vi "Respond.vi"(7 "Sender is Waiting?(F)":bool, 8 "error in (no error)":errorcluster, 9 "Data":refnum<class "Data.lvclass">, 10 "Actor in":refnum<class "Actor.lvclass">, 11 "Request Reply Core in":refnum<class "Request Reply Core.lvclass">) -> (0 "error out":errorcluster, 2 "Actor out":refnum<class "Actor.lvclass">)   [LabVIEW 2020, in "Publisher.lvlib" / "Request Reply Core.lvclass"]
doc: "Handle the Data Action response.\n\nThe default drops the response core and does nothing else."
uses:
  Request Reply Core.lvclass
  PPL/HDH.Data.Generic.lvlibp/Data.lvclass
  PPL/HDH.Actor Framework.Core.Actor.lvlibp/1abvi3w/vi.lib/ActorFramework/Actor/Actor.lvclass
  Request Reply Core.lvclass/Request Reply Core.ctl
  Data/Request Data/Request Data.lvclass/Request Data.ctl
  Data Msg/Data Msg.lvclass/Data Msg.ctl
  Publisher Messages/Addressed Msg/Addressed Msg.lvclass/Addressed Msg.ctl
  Data/Request Data/Request Data.lvclass
  C:/Current projects/WS/PPL/HDH.Data.Generic.lvlibp/Data.lvclass
  Data Msg/Data Msg.lvclass
  C:/Current projects/WS/PPL/HDH.Actor Framework.Core.Actor.lvlibp/1abvi3w/vi.lib/ActorFramework/Message/Message.lvclass
  Publisher Messages/Addressed Msg/Addressed Msg.lvclass
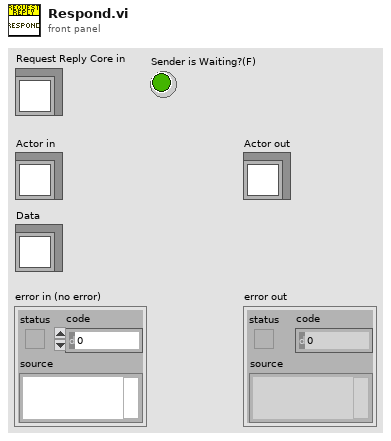
[diagram p1: front panel]
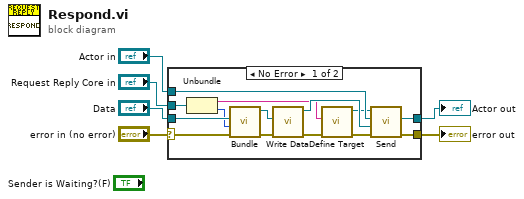
[diagram p0: block diagram]
diagram:
  n1 = case shown="No Error" "error in (no error)" {
    selector: "error in (no error)" -> [w17 w22]
    tunnel: "Request Reply Core in" -> [w20 _]
    tunnel: [w7 w22] -> w4
    tunnel: [w15 w21] -> w3
    tunnel: "Actor in" -> [w16 w21]
    tunnel: "Data" -> [w19 _]
    frame No Error {
      n2 = Unbundle(w20) -> (w11:string, w18:u32)
      n3 = call "Bundle.vi"("error in (no error)"=w17, "Request ID"=w18, "Data"=w19) -> ("error out"=w13:errorcluster, "Request Data out"=w14:refnum<class "Request Data.lvclass">)  [unwired: 7 in]
      n4 = call "Write Data.vi"("error in (no error)"=w13, "Data"=w14) -> ("error out"=w9:errorcluster, "Data Msg out"=w12:refnum<class "Data Msg.lvclass">)  [unwired: 8 in]
      n5 = call "Define Target.vi"("error in (no error)"=w9, "Target Enqueuer ID"=w11) -> ("error out"=w8:errorcluster, "Targetted Msg out"=w10:refnum<class "Addressed Msg.lvclass">)  [unwired: 8 in]
      n6 = call-dynamic "Send.vi"("error in (no error)"=w8, "Message"=w12, "Actor in"=w16, "Addressed Msg in"=w10) -> ("error out"=w7:errorcluster, "Actor out"=w15:refnum<class "Actor.lvclass">)  [unwired: 5 in, 1 out]
    }
    frame Error {
    }
  }
  "error out" <- w4
  "Actor out" <- w3
